vi "Main.vi"() -> ()   [LabVIEW 2015]
doc: "This template is for the Queued Message Handler design pattern.\n\nThe Event Handling Loop generates messages based on user interface actions.\n\nThe Message Handling Loop processes messages generated by the Event Handling Loop, or by other messages. The messages are string values, so new messages can be added easily to the Message Cases case structure in the Message Handling Loop. Each message cluster can also provide an optional value for Message Data, which is a variant that can be converted to whatever message-specific data is required."
uses:
  controls/MCC DAQ Setup.ctl
  support/Message Queue/Message Queue.lvlib
  <vilib>/Utility/error.llb/Error Cluster From Error Code.vi
  support/User Event - Stop/User Event - Stop.lvlib
  support/Message Queue/Enqueue Message (Single).vi
  <vilib>/ErrorRing/Error Ring.xnode
  controls/Aux Sensor.ctl
panel:
  out "Display <Replace Me>":string
  in  "Do Something Else <Replace Me>":bool
  in  "Do Something <Replace Me>":bool
  in  "Exit":bool
  # "These controls have associated \"Value Changed\" events configured in the Event Structure on the diagram.\n\nReplace them (and reconfigure the Event Structure) with the controls you need for your application."
  # "This template is for the Queued Message Handler design pattern.\n\nSee the block diagram for more information on how to use this template."
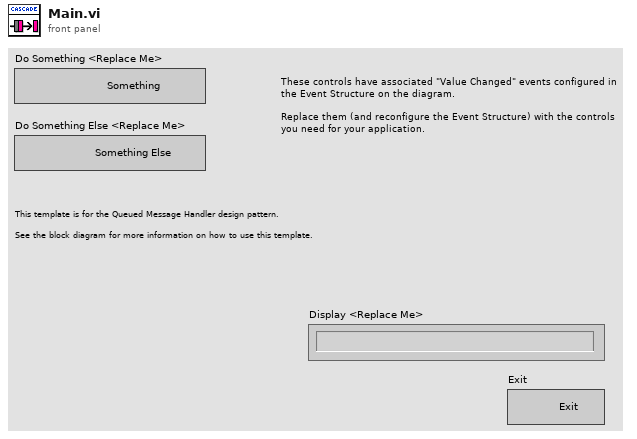
[diagram p1: front panel]
types:
  T1 = typedef "MCC DAQ Setup.ctl" = cluster{"Device Name in InstaCal":string, "Omega Pressure Sensor":T2, "McMillian 102 Flowmeter":T2, "DHT Pressure Sensor":T2, "Top String Pot":T2, "String Pot Signal":T2, "Aux Sensor 1":T2, "Aux Sensor 2":T2, "Aux Sensor 3":T2, "Aux Sensor 4":T2, "Voltage Monitor":T2}
  T2 = typedef "Aux Sensor.ctl" = cluster{"DAQ Channel":dbl, "Output Voltage Range":u16, "Enabled":bool, "Description":string}
  T3 = typedef "Message Queue.lvlib/All Message Queues.ctl" = cluster{"UI":refnum<queue>}
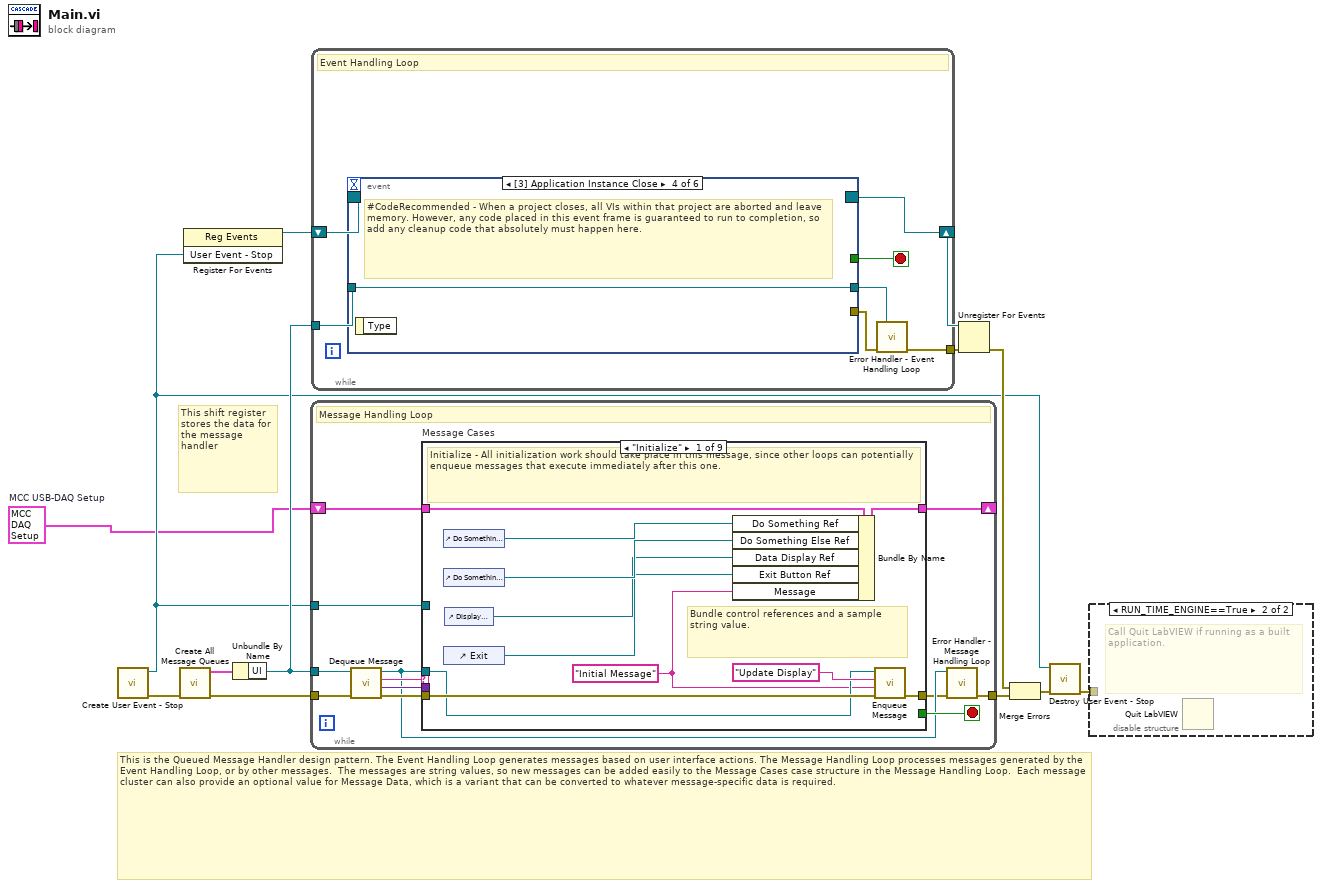
[diagram p0: block diagram]
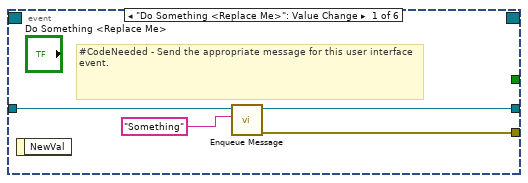
[diagram p3: hidden frame]
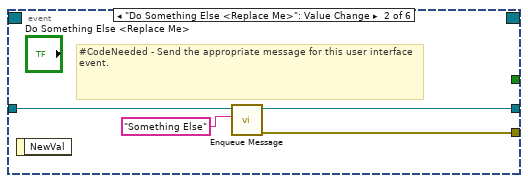
[diagram p4: hidden frame]
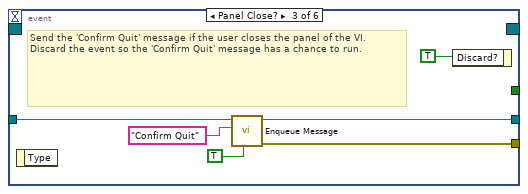
[diagram p5: hidden frame]
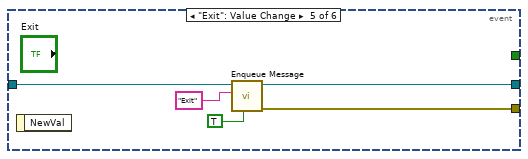
[diagram p6: hidden frame]
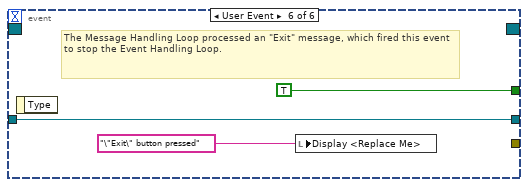
[diagram p7: hidden frame]
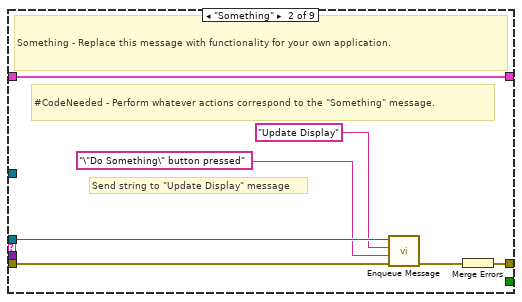
[diagram p8: hidden frame]
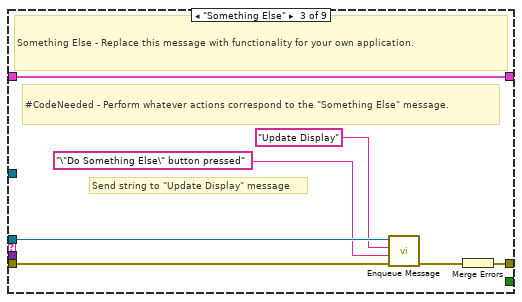
[diagram p9: hidden frame]
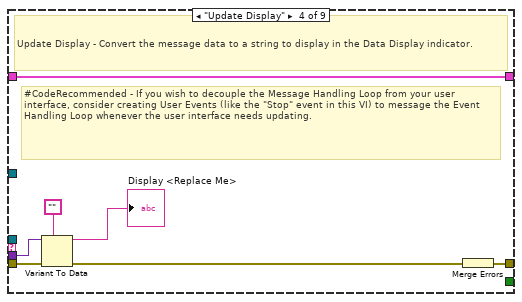
[diagram p10: hidden frame]
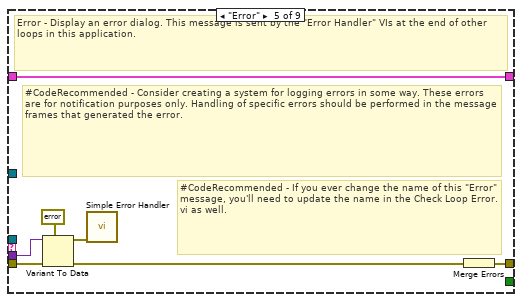
[diagram p11: hidden frame]
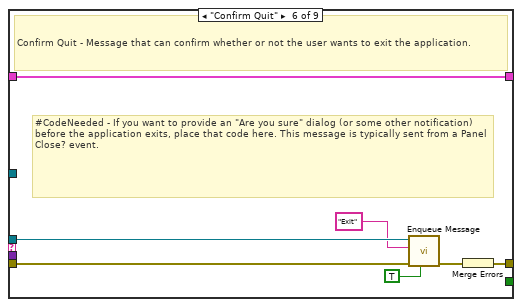
[diagram p12: hidden frame]
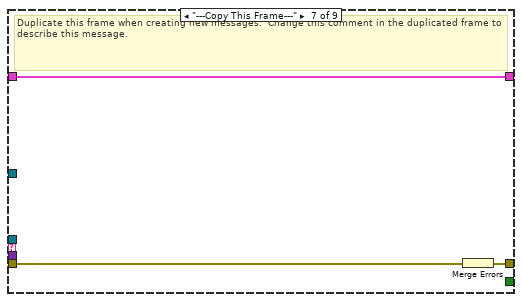
[diagram p13: hidden frame]
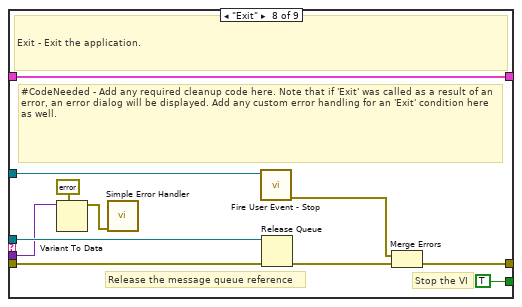
[diagram p14: hidden frame]
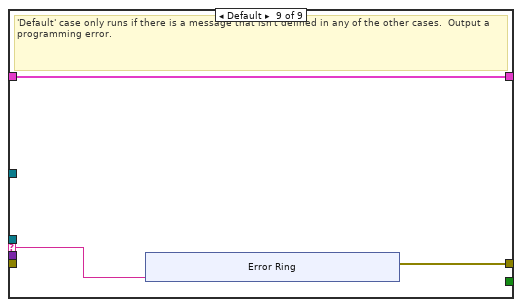
[diagram p15: hidden frame]
diagram:
  w1 = T1 {"Device Name in InstaCal"="Dev0", "Omega Pressure Sensor"={"DAQ Channel"=2.0, "Output Voltage Range"=11, "Enabled"=FALSE, "Description"=""}, "McMillian 102 Flowmeter"={"DAQ Channel"=3.0, "Output Voltage Range"=0, "Enabled"=TRUE, "Description"=""}, "DHT Pressure Sensor"={"DAQ Channel"=1.0, "Output Voltage Range"=5, "Enabled"=TRUE, "Description"=""}, "Top String Pot"={"DAQ Channel"=6.0, "Output Voltage Range"=7, "Enabled"=TRUE, "Description"=""}, "String Pot Signal"={"DAQ Channel"=15.0, "Output Voltage Range"=8, "Enabled"=FALSE, "Description"=""}, "Aux Sensor 1"={"DAQ Channel"=5.0, "Output Voltage Range"=1, "Enabled"=FALSE, "Description"="Aux 1"}, "Aux Sensor 2"={"DAQ Channel"=6.0, "Output Voltage Range"=1, "Enabled"=FALSE, "Description"="Aux 2"}, "Aux Sensor 3"={"DAQ Channel"=7.0, "Output Voltage Range"=1, "Enabled"=TRUE, "Description"="Aux 3"}, "Aux Sensor 4"={"DAQ Channel"=15.0, "Output Voltage Range"=1, "Enabled"=TRUE, "Description"="Aux 4"}, "Voltage Monitor"={"DAQ Channel"=8.0, "Output Voltage Range"=0, "Enabled"=TRUE, "Description"="9V Monitor"}}  # MCC USB-DAQ Setup
  # "This is the Queued Message Handler design pattern. The Event Handling Loop generates messages based on user interface actions. The Message Handling Loop processes messages generated by the Event Handling Loop, or by other messages.  The messages are string values, so new messages can be added easily to the Message Cases case structure in the Message Handling Loop.  Each message cluster can also provide an optional value for Message Data, which is a variant that can be converted to whatever message-specific data is required."
  # "This shift register stores the data for the message handler"
  n1 = call "Create User Event - Stop.vi"() -> ("error out"=w9:errorcluster, "User Event - Stop"=w2:refnum<user-event>)  [unwired: 10 in]
  n2 = call "Create All Message Queues.vi"("error in (no error)"=w9) -> ("error out"=w13:errorcluster, "Message Queues out"=w12:T3)  [unwired: 9 in]
  n3 = register-events(w2) -> (reference out=w3:refnum<event-registration>)  [unwired: 2 in, 1 out]
  n4 = Unbundle By Name(w12) -> ("UI"=w10:refnum<queue>)
  n5 = while {
    tunnel: w10 -> [w17]
    shift-right: [w24] -> _
    shift-left: w1 -> [w25]
    tunnel: w2 -> [w22]
    tunnel: w13 -> [w21]
    tunnel: [w15] -> w11
    stop <- w23 stop-if-true
    # "Message Handling Loop"
    n6 = call "Dequeue Message.vi"("error in (no error)"=w21, "Message Queue"=w17) -> ("error out"=w20:errorcluster, "Message Data"=w18:variant, "Message"=w19:string, "dup Message Queue"=w16:refnum<queue>)  [unwired: 6 in]
    n7 = case "Message Cases" shown="\"Initialize\"" w19 {
      selector: w19 -> [_ _ _ _ _ _ _ _ w86]
      tunnel: w16 -> [w27 w39 w46 _ _ w67 _ w85 _]
      tunnel: w20 -> [w35 w41 w48 w55 w64 w71 w74 w78 _]
      tunnel: [w36 w42 w49 w56 w58 w69 w72 w81 w87] -> w14
      tunnel: w25 -> [w34 w43 w50 w57 w63 w70 w73 w84 w88]
      tunnel: [w33 w43 w50 w57 w63 w70 w73 w84 w88] -> w24
      tunnel: [_ _ _ _ _ _ _ TRUE _] -> w23
      tunnel: w18 -> [_ _ _ w54 w62 _ _ w75 _]
      tunnel: w22 -> [_ _ _ _ _ _ _ w80 _]
      frame "Initialize" {
        w26 = "Initial Message" ("Initial Message")
        # "Bundle control references and a sample string value."
        # "Initialize - All initialization work should take place in this message, since other loops can potentially enqueue messages that execute immediately after this one."
        n8 = control-ref of="Do Something <Replace Me>"() -> (w32:refnum<vi>)
        n9 = control-ref of="Do Something Else <Replace Me>"() -> (w31:refnum<vi>)
        n10 = control-ref of="Exit"() -> (w29:refnum<vi>)
        n11 = control-ref of="Display <Replace Me>"() -> (w30:refnum<vi>)
        n12 = Bundle By Name(cluster=w34, "Do Something Ref"=w32, "Do Something Else Ref"=w31, "Data Display Ref"=w30, "Exit Button Ref"=w29, "Message"=w26) -> (w33:T1)
        n13 = call-poly "Enqueue Message.vi"("error in (no error)"=w35, "Message Data"=w26, "Message"="Update Display", "Message Queue"=w27) -> ("error out"=w36:errorcluster)  [unwired: 6 in, 1 out]
      }
      frame "Something" {
        # "Send string to \"Update Display\" message"
        # "#CodeNeeded - Perform whatever actions correspond to the \"Something\" message."
        # "Something - Replace this message with functionality for your own application."
        n14 = call-poly "Enqueue Message.vi"("error in (no error)"=w41, "Message Data"="\"Do Something\" button pressed" ("\"Do Something\" button pressed"), "Message"="Update Display", "Message Queue"=w39) -> ("error out"=w40:errorcluster)  [unwired: 6 in, 1 out]
        n15 = Merge Errors(w40) -> (w42:errorcluster)
      }
      frame "Something Else" {
        # "Send string to \"Update Display\" message"
        # "#CodeNeeded - Perform whatever actions correspond to the \"Something Else\" message."
        # "Something Else - Replace this message with functionality for your own application."
        n16 = call-poly "Enqueue Message.vi"("error in (no error)"=w48, "Message Data"="\"Do Something Else\" button pressed" ("\"Do Something Else\" button pressed"), "Message"="Update Display", "Message Queue"=w46) -> ("error out"=w47:errorcluster)  [unwired: 6 in, 1 out]
        n17 = Merge Errors(w47) -> (w49:errorcluster)
      }
      frame "Update Display" {
        # "#CodeRecommended - If you wish to decouple the Message Handling Loop from your user interface, consider creating User Events (like the \"Stop\" event in this VI) to message the Event Handling Loop whenever the user interface needs updating."
        # "Update Display - Convert the message data to a string to display in the Data Display indicator."
        n18 = Variant To Data(error in=w55, type="", Variant=w54) -> (data=→"Display <Replace Me>":string, error out=w52:errorcluster)
        n19 = Merge Errors(w52) -> (w56:errorcluster)
      }
      frame "Error" {
        # "#CodeRecommended - If you ever change the name of this \"Error\" message, you'll need to update the name in the Check Loop Error.vi as well."
        # "#CodeRecommended - Consider creating a system for logging errors in some way. These errors are for notification purposes only. Handling of specific errors should be performed in the message frames that generated the error."
        # "Error - Display an error dialog. This message is sent by the \"Error Handler\" VIs at the end of other loops in this application."
        n20 = Variant To Data(error in=w64, type=errorcluster {"status"=FALSE, "code"=0, "source"=""} ("error constant"), Variant=w62) -> (data=w60:errorcluster, error out=w59:errorcluster)
        n21 = call <vilib>:"Simple Error Handler.vi"("error in (no error)"=w60) -> ()  [unwired: 4 in, 5 out]
        n22 = Merge Errors(w59) -> (w58:errorcluster)
      }
      frame "Confirm Quit" {
        # "#CodeNeeded - If you want to provide an \"Are you sure\" dialog (or some other notification) before the application exits, place that code here. This message is typically sent from a Panel Close? event."
        # "Confirm Quit - Message that can confirm whether or not the user wants to exit the application."
        n23 = call-poly "Enqueue Message.vi"("Priority Message? (F)"=TRUE, "error in (no error)"=w71, "Message"="Exit", "Message Queue"=w67) -> ("error out"=w68:errorcluster)  [unwired: 6 in, 1 out]
        n24 = Merge Errors(w68) -> (w69:errorcluster)
      }
      frame "---Copy This Frame---" {
        # "Duplicate this frame when creating new messages.  Change this comment in the duplicated frame to describe this message."
        n25 = Merge Errors(w74) -> (w72:errorcluster)
      }
      frame "Exit" {
        # "Stop the VI"
        # "Release the message queue reference"
        # "#CodeNeeded - Add any required cleanup code here. Note that if 'Exit' was called as a result of an error, an error dialog will be displayed. Add any custom error handling for an 'Exit' condition here as well."
        # "Exit - Exit the application."
        n26 = Variant To Data(type=errorcluster {"status"=FALSE, "code"=0, "source"=""} ("error constant"), Variant=w75) -> (data=w76:errorcluster)  [unwired: 1 in, 1 out]
        n27 = call <vilib>:"Simple Error Handler.vi"("error in (no error)"=w76) -> ()  [unwired: 4 in, 5 out]
        n28 = call "Fire User Event - Stop.vi"("User Event - Stop"=w80) -> ("error out"=w79:errorcluster)  [unwired: 10 in]
        n29 = Release Queue(queue=w85, error in (no error)=w78) -> (error out=w82:errorcluster)  [unwired: 1 in, 2 out]
        n30 = Merge Errors(w79, w82) -> (w81:errorcluster)
      }
      frame Default {
        # "'Default' case only runs if there is a message that isn't defined in any of the other cases.  Output a programming error."
        n31 = xnode "Error Ring"("parameter 0"=w86) -> ("error out"=w87:errorcluster)
      }
    }
    n32 = call "Error Handler - Message Handling Loop.vi"("error in (no error)"=w14, "Message Queue"=w16) -> ("dup error in"=w15:errorcluster)  [unwired: 8 in, 1 out]
  }
  n33 = while {
    tunnel: w10 -> [w102]
    shift-right: [w100] -> w6
    shift-left: w3 -> [w101]
    tunnel: [w96] -> w4
    stop <- w98 stop-if-true
    # "Event Handling Loop"
    n34 = event shown="[3] Application Instance Close" {
      selector: w101 -> [_ _ _ _ _ _]
      dyn-events: [_ _ _ _ _ _] -> w100
      timeout: _ -> [_ _ _ _ _ _]
      tunnel: [_ _ _ _ _ TRUE ("Discard?")] -> w98
      tunnel: w102 -> [w106 w110 w115 w117 w122 w125]
      tunnel: [w103 w107 w114 _ w121 _] -> w99
      tunnel: [w105 w109 w113 w117 w120 w125] -> w97
      event "Do Something <Replace Me>": Value Change {
        # "#CodeNeeded - Send the appropriate message for this user interface event."
        n35 = event-data() -> ()  [unwired: 1 in, 1 out]
        n36 = call-poly "Enqueue Message.vi"("Message"="Something", "Message Queue"=w106) -> ("error out"=w103:errorcluster, "dup Message Queue"=w105:refnum<queue>)  [unwired: 8 in]
      }
      event "Do Something Else <Replace Me>": Value Change {
        # "#CodeNeeded - Send the appropriate message for this user interface event."
        n37 = event-data() -> ()  [unwired: 1 in, 1 out]
        n38 = call-poly "Enqueue Message.vi"("Message"="Something Else", "Message Queue"=w110) -> ("error out"=w107:errorcluster, "dup Message Queue"=w109:refnum<queue>)  [unwired: 8 in]
      }
      event Panel Close? {
        # "Send the 'Confirm Quit' message if the user closes the panel of the VI. Discard the event so the 'Confirm Quit' message has a chance to run."
        n39 = event-data() -> ()  [unwired: 1 in, 1 out]
        n40 = call-poly "Enqueue Message.vi"("Priority Message? (F)"=TRUE, "Message"="Confirm Quit", "Message Queue"=w115) -> ("error out"=w114:errorcluster, "dup Message Queue"=w113:refnum<queue>)  [unwired: 7 in]
        n41 = event-data("Discard?"=TRUE) -> ()  [unwired: 1 in, 1 out]
      }
      event Application Instance Close {
        # "#CodeRecommended - When a project closes, all VIs within that project are aborted and leave memory. However, any code placed in this event frame is guaranteed to run to completion, so add any cleanup code that absolutely must happen here."
        n42 = event-data() -> ()  [unwired: 1 in, 1 out]
      }
      event "Exit": Value Change {
        n43 = event-data() -> ()  [unwired: 1 in, 1 out]
        n44 = call-poly "Enqueue Message.vi"("Priority Message? (F)"=TRUE, "Message"="Exit", "Message Queue"=w122) -> ("error out"=w121:errorcluster, "dup Message Queue"=w120:refnum<queue>)  [unwired: 7 in]
      }
      event User Event {
        # "The Message Handling Loop processed an \"Exit\" message, which fired this event to stop the Event Handling Loop."
        n45 = event-data() -> ()  [unwired: 1 in, 1 out]
        n46 = local write "Display <Replace Me>"("\"Exit\" button pressed" ("VI Stopped")) -> ()
      }
    }
    n47 = call "Error Handler - Event Handling Loop.vi"("error in (no error)"=w99, "Message Queue"=w97) -> ("dup error in"=w96:errorcluster)  [unwired: 8 in, 1 out]
  }
  n48 = Unregister For Events(event registration refnum=w6, error in=w4) -> (error out=w7:errorcluster)
  n49 = Merge Errors(w7, w11) -> (w8:errorcluster)
  n50 = call "Destroy User Event - Stop.vi"("error in (no error)"=w8, "User Event - Stop"=w2) -> ("error out"=w5:errorcluster)  [unwired: 9 in]
  n51 = disable-structure shown="RUN_TIME_ENGINE==True" {
    disable-tunnel: w5 -> [_ _]
    frame condition #0 (active) {
    }
    frame condition #1 {
      # "Call Quit LabVIEW if running as a built application."
      n52 = Quit LabVIEW() -> ()  [unwired: 1 in]
    }
  }
